vi "推拉力判定.vi"(7 "Result":refnum<vi>, 10 "判定参数":T1={"角度调节最大力"={"单位"="N", "下限"=3.0, "上限"=4.0}}, 11 "XY曲线":cluster{"X":dbl[], "Y":dbl[]}[](array[cluster])) -> (2 "判定项长度":i32, 3 "OK？":bool)   [LabVIEW 2020]
panel:
  out "转置的数组":string[][](array[string])
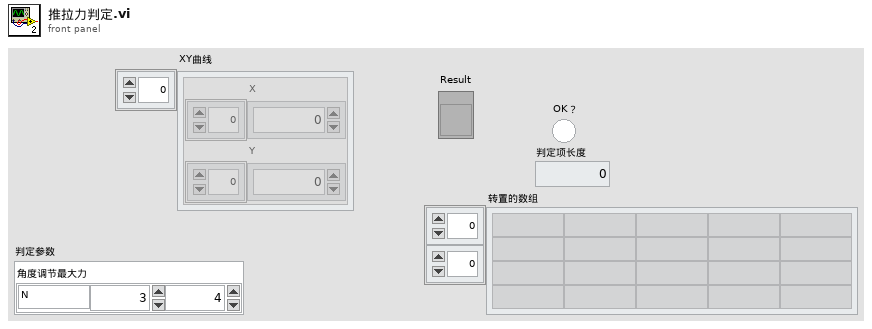
[diagram p1: front panel]
types:
  T1 = cluster{"角度调节最大力":cluster{"单位":string, "下限":dbl, "上限":dbl}}
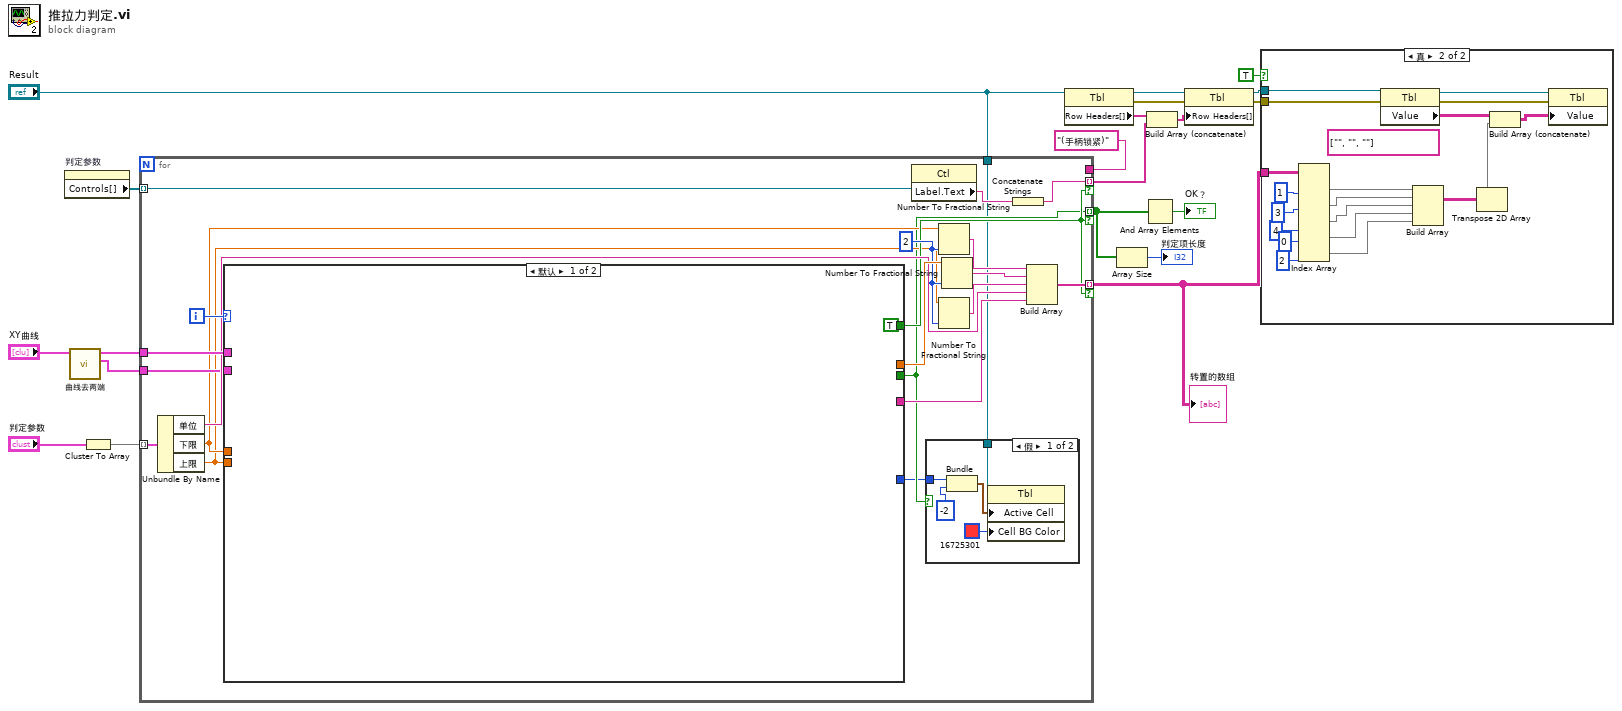
[diagram p0: block diagram]
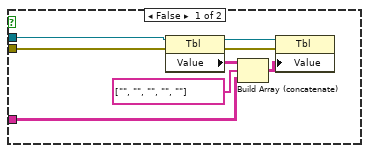
[diagram p2: hidden frame]
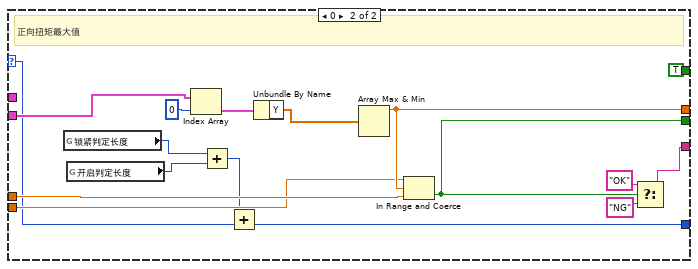
[diagram p4: hidden frame]
diagram:
  n1 = property on="判定参数" class="Clust (严格)"() -> ("Controls[]"=w12:refnum<vi>[])  [unwired: 2 in, 2 out]
  n2 = call "曲线去两端.vi"("曲线In"="XY曲线") -> ("启动曲线"=w5:cluster{"X":dbl[], "Y":dbl[]}[], "曲线Out"=w8:cluster{"X":dbl[], "Y":dbl[]}[])  [unwired: 9 in]
  n3 = Cluster To Array(cluster="判定参数") -> (array=w2:cluster{"单位":string, "下限":dbl, "上限":dbl}[])
  n4 = for {
    tunnel: w12 -> [w40] mode=indexing
    tunnel: w8 -> [w38]
    tunnel: [w23] -> w7 mode=indexing if=w29
    tunnel: [w31] -> w3 mode=indexing if=w29
    tunnel: [w25] -> w14 mode=indexing if=w29
    tunnel: w5 -> [w28]
    tunnel: "(手柄锁紧)" ("Label.Text") -> [_]
    tunnel: w2 -> [w24] mode=indexing
    tunnel: "Result" -> [w22]
    i -> [w41]
    w37 = i16 2 ("精度(6)")
    n5 = Unbundle By Name(w24) -> ("单位"=w32:string, "下限"=w27:dbl, "上限"=w26:dbl)
    n6 = case shown="默认" w41 {
      selector: w41 -> [_ w52]
      tunnel: [_ w62] -> w39
      tunnel: w38 -> [_ _]
      tunnel: [_ w59] -> w33
      tunnel: [_ w58] -> w23
      tunnel: w27 -> [_ w57]
      tunnel: w26 -> [_ w56]
      tunnel: [TRUE TRUE] -> w29
      tunnel: w28 -> [_ w53]
      tunnel: [_ w51] -> w21
      frame Default {
      }
      frame 0 {
        # "正向扭矩最大值"
        n7 = global read "判定参数.vi" "锁紧判定长度"() -> (w50:i32)
        n8 = global read "判定参数.vi" "开启判定长度"() -> (w49:i32)
        n9 = Index Array(array=w53, index=0 ("索引")) -> (element=w63:cluster{"X":dbl[], "Y":dbl[]})
        n10 = Add(x=w50, y=w49) -> (x+y=w48:i32)
        n11 = Add(x=w48, y=w52) -> (x+y=w51:i32)
        n12 = Unbundle By Name(w63) -> ("Y"=w54:dbl[])
        n13 = Array Max & Min(array=w54) -> (max value=w62:dbl)  [unwired: 3 out]
        n14 = In Range and Coerce(upper limit=w56, x=w62, lower limit=w57) -> (In Range?=w58:bool)  [unwired: 1 out]
        n15 = Select(t="OK", s=w58, f="NG") -> (s? t:f=w59:string)
      }
    }
    n16 = property class="Ctl"(reference=w40) -> ("Label.Text"=w30:string)  [unwired: 1 in, 2 out]
    n17 = case shown="假" w23 {
      tunnel: w22 -> [w46 _]
      tunnel: w21 -> [w44 _]
      frame False {
        n18 = Bundle(w44, "索引"=-2) -> (w42:cluster{i32, "索引":i32})  [unwired: 1 in]
        n19 = property class="Tbl"(reference=w46, "Active Cell"=w42, "Cell BG Color"=u32 16725301 ("活动单元格:单元格背景色")) -> ()  [unwired: 1 in, 2 out]
      }
      frame True {
      }
    }
    n20 = Number To Fractional String(number=w27, precision (6)=w37) -> (F-format string=w36:string)  [unwired: 2 in]
    n21 = Number To Fractional String(number=w26, precision (6)=w37) -> (F-format string=w34:string)  [unwired: 2 in]
    n22 = Number To Fractional String(number=w39, precision (6)=w37) -> (F-format string=w35:string)  [unwired: 2 in]
    n23 = Concatenate Strings(w30) -> (w25:string)
    n24 = Build Array(w36, w35, w34, w32, w33) -> (w31:string[])
  }
  "转置的数组" <- w3
  n25 = property class="Tbl"(reference="Result") -> (reference out=w16:refnum<vi>, error out=w19:errorcluster, "Row Headers[]"=w13:string[])  [unwired: 1 in]
  n26 = Array Size(array=w7) -> (size(s)=→"判定项长度":i32)
  n27 = And Array Elements(Boolean array=w7) -> (logical AND=→"OK？":bool)
  n28 = Build Array (concatenate)(w13, w14) -> (w15:string[])
  n29 = property class="Tbl"(reference=w16, error in=w19, "Row Headers[]"=w15) -> (reference out=w17:refnum<vi>, error out=w18:errorcluster)
  n30 = case shown="真" TRUE {
    tunnel: w18 -> [w70 w90]
    tunnel: w17 -> [w67 w87]
    tunnel: w3 -> [w66 w84]
    frame False {
      n31 = property class="Tbl"(reference=w67, error in=w70) -> (reference out=w68:refnum<vi>, error out=w69:errorcluster, "Value"=w71:string[][])
      n32 = Build Array (concatenate)(w71, string[] ["", "", "", "", ""], w66) -> (w72:string[][])
      n33 = property class="Tbl"(reference=w68, error in=w69, "Value"=w72) -> ()  [unwired: 2 out]
    }
    frame True {
      (unwired) string[] ["", "", ""]
      n34 = Index Array(array=w84, index (col) #1=1 ("禁用的索引 (列)"), index (col) #2=3 ("索引 (列)"), index (col) #3=4 ("索引 (列)"), index (col) #4=0 ("索引 (列)"), index (col) #5=2 ("索引 (列)")) -> (element #1=w79:string[], element #2=w78:string[], element #3=w77:string[], element #4=w76:string[], element #5=w75:string[])  [unwired: 5 in]
      n35 = property class="Tbl"(reference=w87, error in=w90) -> (reference out=w88:refnum<vi>, error out=w89:errorcluster, "Value"=w91:string[][])
      n36 = Build Array(w79, w78, w77, w76, w75) -> (w81:string[][])
      n37 = Transpose 2D Array ("二维数组转置")(2D array=w81) -> (transposed array=w73:string[][])
      n38 = Build Array (concatenate)(w91, w73) -> (w80:string[][])
      n39 = property class="Tbl"(reference=w88, error in=w89, "Value"=w80) -> ()  [unwired: 2 out]
    }
  }
